vi "Estructuras de repeticion.vi"() -> ()   [LabVIEW 2011]
panel:
  out "NUMERO":dbl
  in  "DETENER":bool
  # "Estructuras de Repeticion"
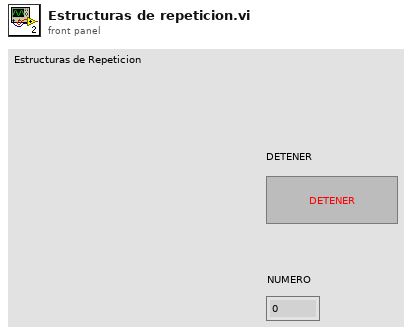
[diagram p1: front panel]
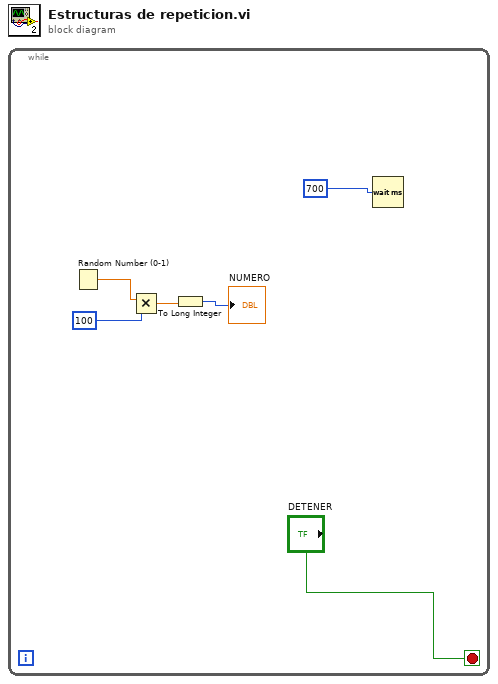
[diagram p0: block diagram]
diagram:
  n1 = while {
    stop <- "DETENER" stop-if-true
    n2 = Random Number (0-1)() -> (number: 0 to 1=w3:dbl)
    n3 = Multiply(x=w3, y=100) -> (x*y=w4:dbl)
    n4 = To Long Integer(number=w4) -> (32bit integer=→"NUMERO":i32)
    n5 = Wait (ms)(milliseconds to wait=700) -> ()  [unwired: 1 out]
  }
